vi "P-541 Stage Engine.vi"(0 "Notifier Name":string, 11 "COM Port":string[](array[string])) -> ()   [LabVIEW 2016]
uses:
  Stages Controls/Stage Focus Control.ctl
  Stages Controls/Stage Status.ctl
  Stages Controls/Stage Notifier Element.ctl
  Stages Controls/Stage Actions.ctl
panel:
  out "x-y":dbl[](array[numeric])
  out "On Target?":bool[](array[boolean])
  out "Positions":dbl[](array[numeric])
  in  "Get Position":bool
  in  "ReInitialize":bool
  in  "Error":bool
  out "Status":T1
  in  "Quit":bool
  in  "Focus Control":T2
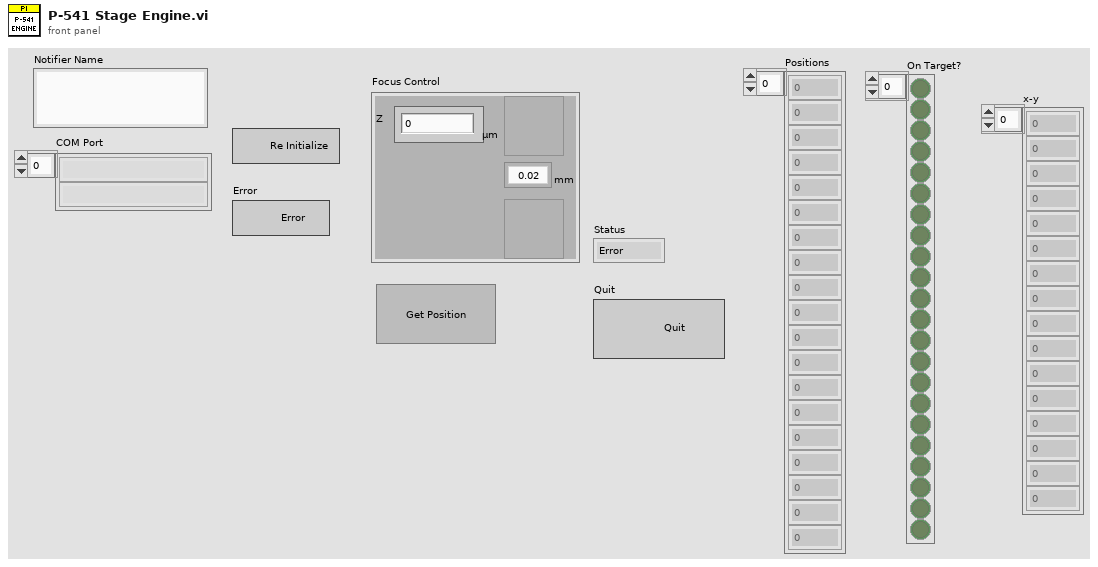
[diagram p1: front panel]
types:
  T1 = typedef "Stage Status.ctl" = enum16{"Error", "Abort", "Busy", "On Target"}
  T2 = typedef "Stage Focus Control.ctl" = cluster{"Focus Step (um)":enum16{"0.02", "0.05", "0.1", "0.5", "1", "2", "5", "10", "20"}, "Focus Up":bool, "Focus Down":bool, "Z ":dbl}
  T3 = typedef "Stage Notifier Element.ctl" = cluster{"Action":T4, "Axis":bool[], "Setpoint":dbl[], "Velocity":dbl, "Cmd Recvd?":bool, "Position":dbl[], "Status":T1, "Misc":variant}
  T4 = typedef "Stage Actions.ctl" = enum16{"Get Position", "MVR", "MOVE", "HALT", "ONTARGET", "ERROR", "REFERENCE", "INIT", "VELOCITY", "STATUS", "EXIT", "HOME", "ZEROPOS", "NANOPOS", "ANALOG", "QUIT"}
  T5 = cluster{"Focus Step (um)":bool, "Focus Up":bool, "Focus Down":bool, "Z ":bool}
  T6 = enum16{"0.02", "0.05", "0.1", "0.5", "1", "2", "5", "10", "20"}
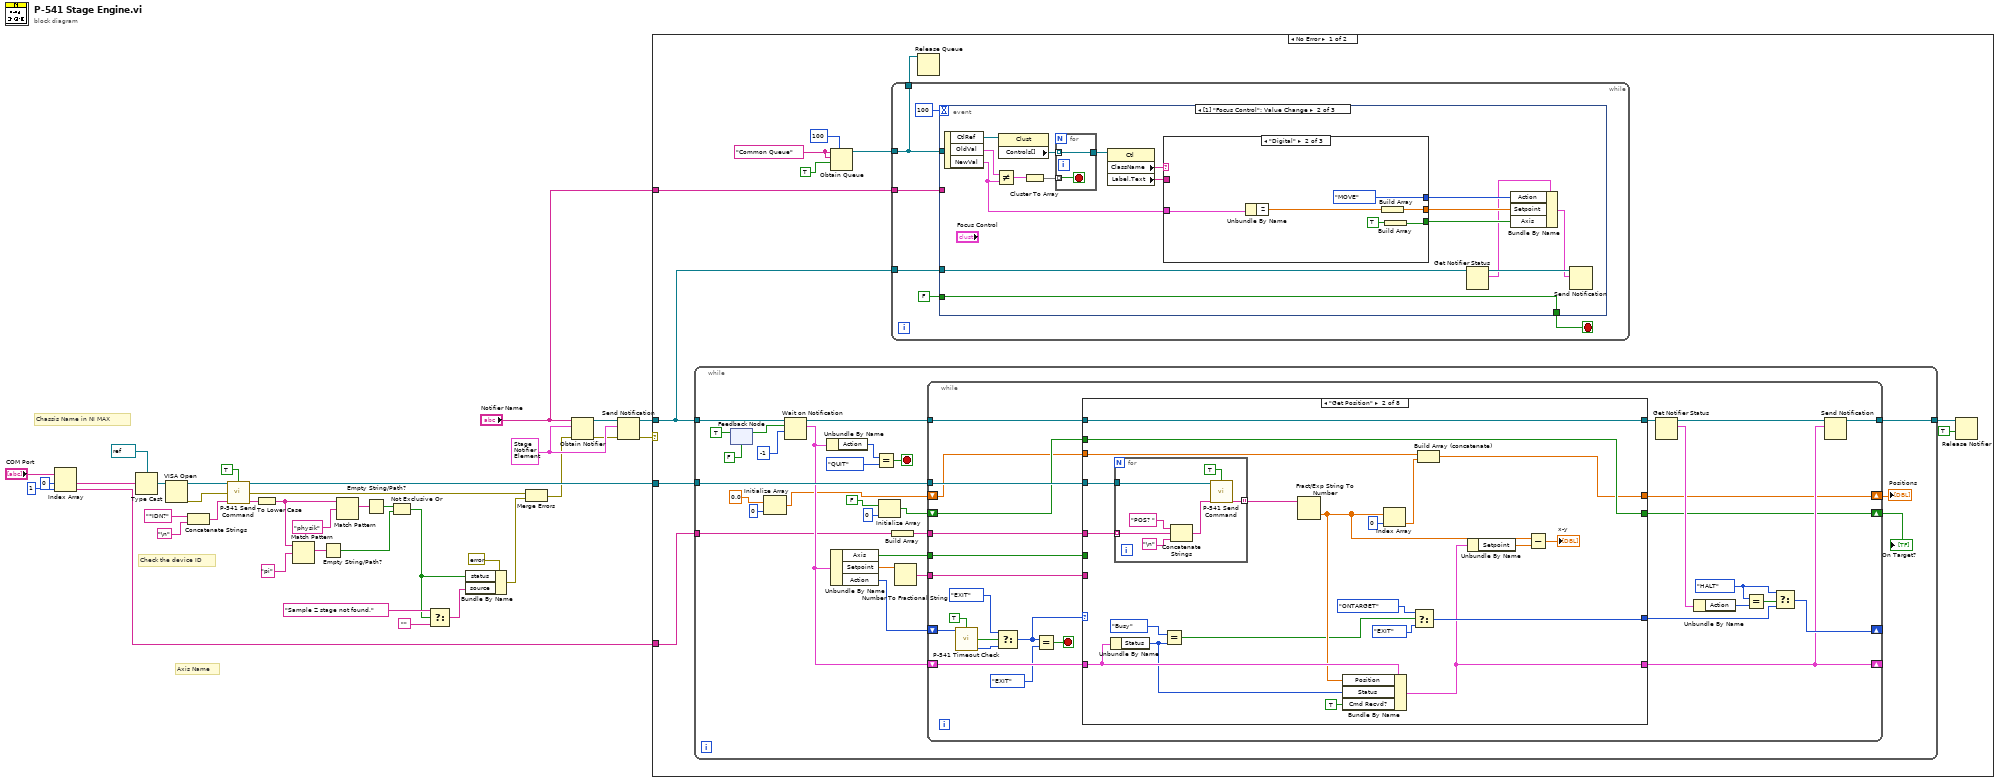
[diagram p0: block diagram]
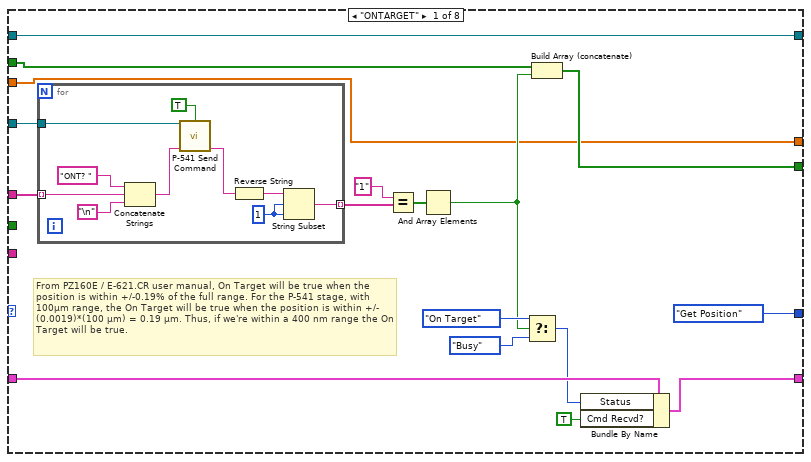
[diagram p2: hidden frame]
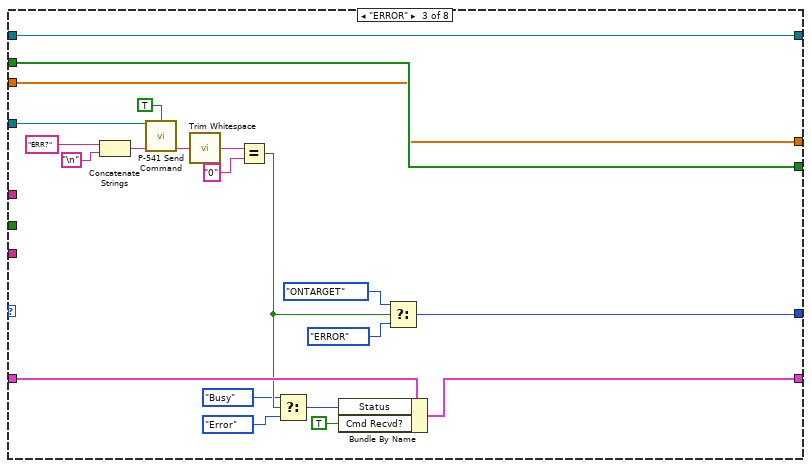
[diagram p3: hidden frame]
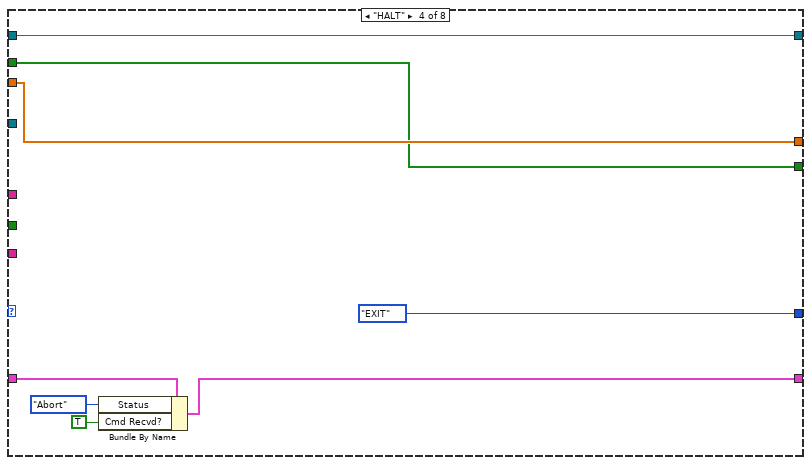
[diagram p4: hidden frame]
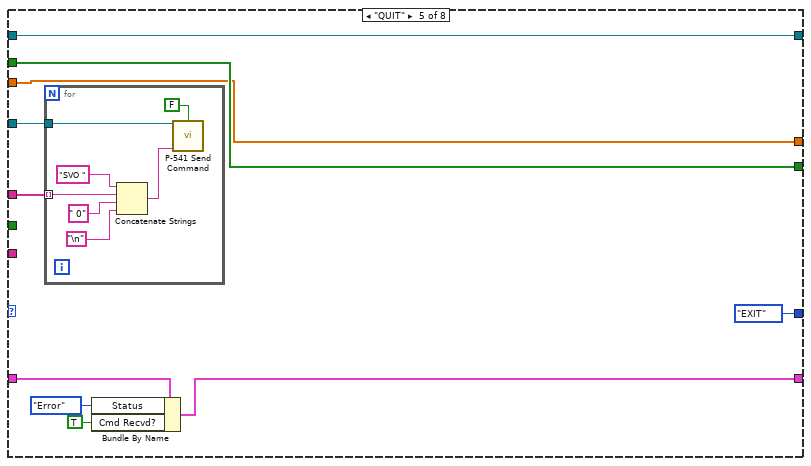
[diagram p5: hidden frame]
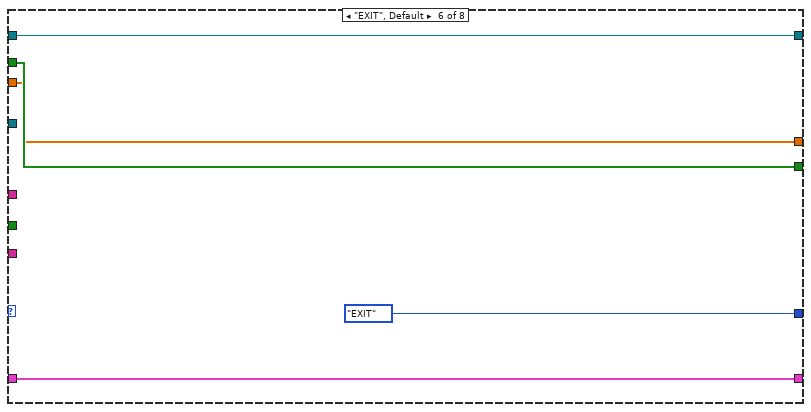
[diagram p6: hidden frame]
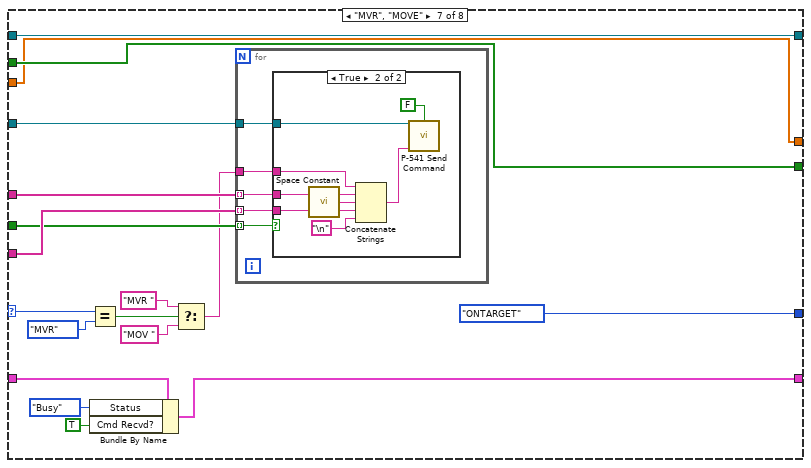
[diagram p7: hidden frame]
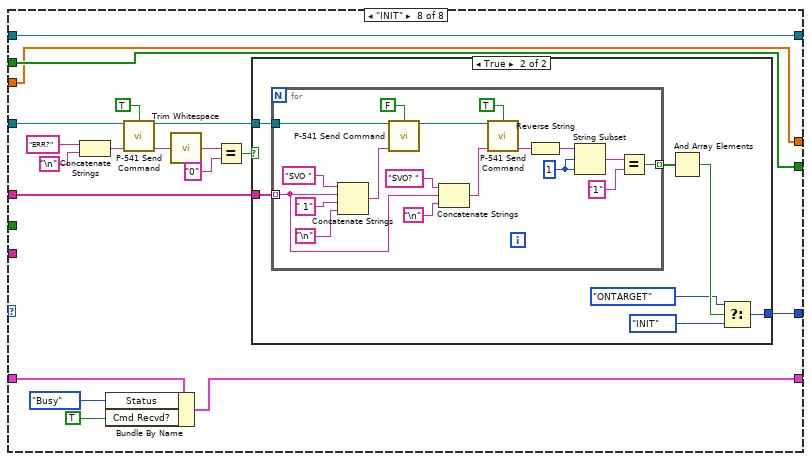
[diagram p9: hidden frame]
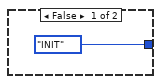
[diagram p10: hidden frame]
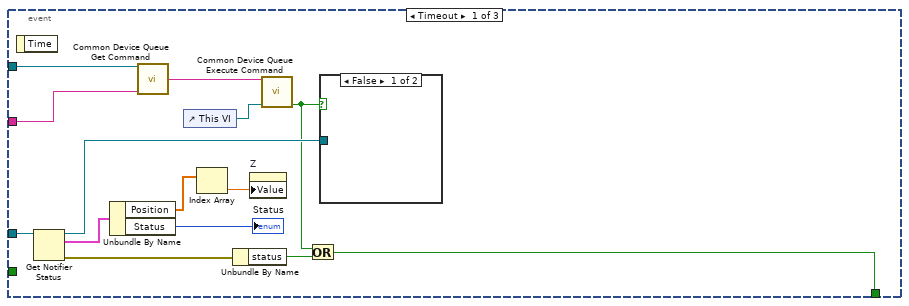
[diagram p11: hidden frame]
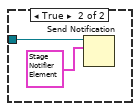
[diagram p12: hidden frame]
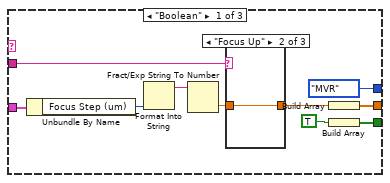
[diagram p13: hidden frame]
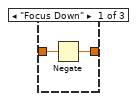
[diagram p14: hidden frame]
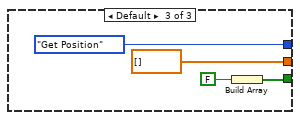
[diagram p16: hidden frame]
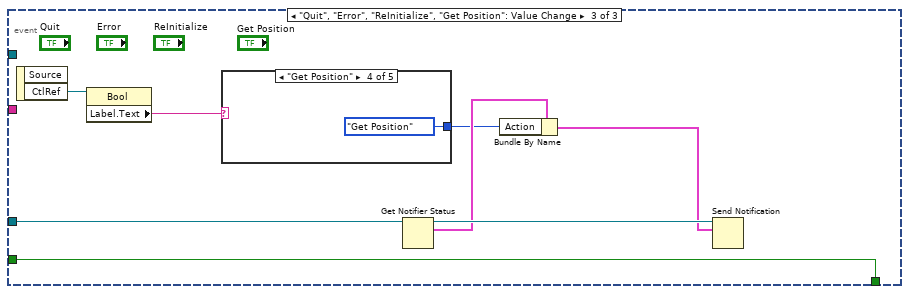
[diagram p17: hidden frame]
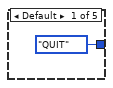
[diagram p18: hidden frame]
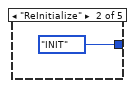
[diagram p19: hidden frame]
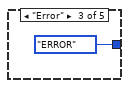
[diagram p20: hidden frame]
diagram:
  w32 = T3 {"Action"=enum."INIT", "Axis"=[], "Setpoint"=[], "Velocity"=0.5, "Cmd Recvd?"=FALSE, "Position"=[], "Status"=enum."Busy", "Misc"=variant} ("Stage Status")
  # "Check the device ID"
  # "Axis Name"
  # "Chassis Name in NI MAX"
  n1 = Index Array(array="COM Port", index #1=0 ("index"), index #2=1 ("index")) -> (element #1=w35:string, element #2=w25:string)
  n2 = Type Cast(type=refnum<visa-resource-name> refnum ("reference out"), x=w35) -> (*(type *) &x=w11:refnum<visa-resource-name>)
  n3 = VISA Open(VISA resource name=w11) -> (VISA resource name=w10:refnum<visa-resource-name>, error out=w7:errorcluster)  [unwired: 4 in]
  n4 = Concatenate Strings("*IDN?" ("string"), "\n") -> (w24:string)
  n5 = call "P-541 Send Command.vi"("VISA Ref"=w10, "Wait for Reply?"=TRUE, "Error In"=w7, "Command"=w24) -> ("VISA Ref Out"=w9:refnum<visa-resource-name>, "Error Out"=w16:errorcluster, "Response"=w18:string)  [unwired: 9 in]
  n6 = To Lower Case(string=w18) -> (all lower case string=w4:string)
  n7 = Match Pattern(string=w4, regular expression="pi" ("string")) -> (match substring=w6:string)  [unwired: 1 in, 3 out]
  n8 = Empty String/Path?(string/path=w6) -> (empty?=w2:bool)
  n9 = Match Pattern(string=w4, regular expression="physik" ("string")) -> (match substring=w20:string)  [unwired: 1 in, 3 out]
  n10 = Empty String/Path?(string/path=w20) -> (empty?=w3:bool)
  n11 = Not Exclusive Or(1:w2, 2:w3) -> (0:w1:bool)
  n12 = Select(t="Sample Z stage not found." ("string"), s=w1, f="") -> (s? t:f=w14:string)
  n13 = Bundle By Name(cluster=errorcluster {"status"=FALSE, "code"=0, "source"=""} ("Error Out"), "status"=w1, "source"=w14) -> (w15:errorcluster)
  n14 = Merge Errors(w16, w15) -> (w8:errorcluster)
  n15 = Obtain Notifier(name (unnamed)="Notifier Name", notification data type=w32, error in (no error)=w8) -> (notifier out=w33:refnum<notifier>, error out=w31:errorcluster)  [unwired: 1 in, 1 out]
  n16 = Send Notification(notification=w32, notifier=w33, error in (no error)=w31) -> (notifier out=w29:refnum<notifier>, error out=w30:errorcluster)
  n17 = case shown="No Error" w30 {
    selector: w30 -> [_ w362]
    tunnel: w29 -> [w41 w364]
    tunnel: w9 -> [w42 w363]
    tunnel: "Notifier Name" -> [w40 _]
    tunnel: w25 -> [w37 _]
    frame No Error {
      w45 = "Common Queue" ("Unique Notifier Name")
      n18 = while {
        tunnel: w41 -> [w72]
        tunnel: w42 -> [w64]
        tunnel: [w57] -> w38
        tunnel: w37 -> [w56]
        stop <- w73 stop-if-true
        n19 = feedback #1(FALSE) -> (w58:bool)
        n20 = feedback-in #1(TRUE) -> ()
        n21 = Initialize Array(0.0, 0 ("dimension size")) -> (w50:dbl[])
        n22 = Wait on Notification(notifier=w72, ignore previous (F)=w58, timeout in ms (-1)=-1) -> (notifier out=w63:refnum<notifier>, notification=w62:T3)  [unwired: 1 in, 2 out]
        n23 = Unbundle By Name(w62) -> ("Action"=w71:T4)
        n24 = Unbundle By Name(w62) -> ("Axis"=w67:bool[], "Setpoint"=w68:dbl[], "Action"=w69:T4)
        n25 = Equal?(x=w71, y=Stage_Actions."QUIT") -> (x = y?=w73:bool)
        n26 = Initialize Array(FALSE, 0 ("dimension size")) -> (w53:bool[])
        n27 = Build Array(w56) -> (w65:string[])
        n28 = Number To Fractional String(number=w68) -> (F-format string=w66:string[])  [unwired: 3 in]
        n29 = while {
          tunnel: w65 -> [w101]
          shift-right: [w82] -> _
          shift-left: w69 -> [w93]
          tunnel: w67 -> [w98]
          tunnel: w66 -> [w99]
          shift-right: [w81] -> _
          shift-left: w62 -> [w97]
          tunnel: w64 -> [w100]
          tunnel: w63 -> [w79]
          tunnel: [w78] -> w57
          shift-right: [w76] -> w48
          shift-left: w53 -> [w77]
          shift-right: [w74] -> w49
          shift-left: w50 -> [w75]
          stop <- w95 stop-if-true
          w84 = Stage_Actions."HALT" ("Action")
          n30 = call "P-541 Timeout Check.vi"("Action"=w93, "User Input?"=TRUE) -> ("Timeout?"=w92:bool, "Action (Dup)"=w91:T4)  [unwired: 12 in]
          n31 = Select(t=Stage_Actions."EXIT" ("y"), s=w92, f=w91) -> (s? t:f=w89:T4)
          n32 = Equal?(x=w89, y=Stage_Actions."EXIT") -> (x = y?=w95:bool)
          n33 = case shown="\"Get Position\"" w89 {
            selector: w89 -> [_ _ _ _ _ _ w216 _]
            tunnel: w101 -> [w118 w149 _ _ w193 _ w225 w257]
            tunnel: w100 -> [w114 w148 w163 _ w194 _ w224 w245]
            tunnel: w99 -> [_ _ _ _ _ _ w223 _]
            tunnel: w98 -> [_ _ _ _ _ _ w222 _]
            tunnel: [Stage_Actions."Get Position" ("y") w146 w172 Stage_Actions."EXIT" ("y") Stage_Actions."EXIT" ("y") Stage_Actions."EXIT" ("y") Stage_Actions."ONTARGET" ("y") w253] -> w83
            tunnel: w97 -> [w111 w144 w167 w181 w191 w207 w219 w254]
            tunnel: [w112 w134 w168 w182 w189 w207 w218 w247] -> w81
            tunnel: [w106 w139 w159 w180 w188 w205 w210 w241] -> w80
            tunnel: w79 -> [w106 w139 w159 w180 w188 w205 w210 w241]
            tunnel: w77 -> [w105 w138 w158 w178 w187 w204 w209 w240]
            tunnel: [w103 w138 w158 w178 w187 w204 w209 w240] -> w76
            tunnel: w75 -> [w102 w136 w157 w179 w186 w203 w208 w239]
            tunnel: [w102 w135 w157 w179 w186 w203 w208 w239] -> w74
            frame "ONTARGET" {
              # "From PZ160E / E-621.CR user manual, On Target will be true when the position is within +/-0.19% of the full range. For the P-541 stage, with 100µm range, the On Target will be true when the position is within +/- (0.0019)*(100 µm) = 0.19 µm. Thus, if we're within a 400 nm range the On Target will be true."
              n34 = for {
                tunnel: w118 -> [w128] mode=indexing
                tunnel: [w127] -> w117 mode=indexing
                tunnel: w114 -> [w121]
                w123 = 1 ("length (rest)")
                n35 = Concatenate Strings("ONT? " ("string"), w128, "\n") -> (w120:string)
                n36 = call "P-541 Send Command.vi"("VISA Ref"=w121, "Wait for Reply?"=TRUE, "Command"=w120) -> ("Response"=w119:string)  [unwired: 10 in, 2 out]
                n37 = Reverse String(1:w119) -> (0:w124:string)
                n38 = String Subset(string=w124, offset (0)=w123, length (rest)=w123) -> (substring=w127:string)
              }
              n39 = Equal?(x="1", y=w117) -> (x = y?=w115:bool[])
              n40 = And Array Elements(Boolean array=w115) -> (logical AND=w104:bool)
              n41 = Select(t=Stage_Status."On Target" ("Status"), s=w104, f=Stage_Status."Busy" ("Status")) -> (s? t:f=w108:T1)
              n42 = Build Array (concatenate)(w105, w104) -> (w103:bool[])
              n43 = Bundle By Name(cluster=w111, "Status"=w108, "Cmd Recvd?"=TRUE) -> (w112:T3)
            }
            frame "Get Position" {
              n44 = Unbundle By Name(w144) -> ("Status"=w142:T1)
              n45 = for {
                tunnel: w149 -> [w156] mode=indexing
                tunnel: w148 -> [w152]
                tunnel: [w150] -> w147 mode=indexing
                n46 = Concatenate Strings("POS? " ("string"), w156, "\n") -> (w151:string)
                n47 = call "P-541 Send Command.vi"("VISA Ref"=w152, "Wait for Reply?"=TRUE, "Command"=w151) -> ("Response"=w150:string)  [unwired: 10 in, 2 out]
              }
              n48 = Equal?(x=Stage_Status."Busy", y=w142) -> (x = y?=w129:bool)
              n49 = Fract/Exp String To Number(string=w147) -> (number=w131:dbl[])  [unwired: 3 in, 1 out]
              n50 = Bundle By Name(cluster=w144, "Position"=w131, "Status"=w142, "Cmd Recvd?"=TRUE) -> (w134:T3)
              n51 = Index Array(array=w131, index=0) -> (element=w133:dbl)
              n52 = Select(t=Stage_Actions."ONTARGET" ("y"), s=w129, f=Stage_Actions."EXIT" ("y")) -> (s? t:f=w146:T4)
              n53 = Build Array (concatenate)(w136, w133) -> (w135:dbl[])
              n54 = Unbundle By Name(w134) -> ("Setpoint"=w132:dbl[])
              n55 = Subtract(x=w131, y=w132) -> (x-y=→"x-y":dbl[])
            }
            frame "ERROR" {
              n56 = Concatenate Strings("ERR?" ("string"), "\n") -> (w162:string)
              n57 = call "P-541 Send Command.vi"("VISA Ref"=w163, "Wait for Reply?"=TRUE, "Command"=w162) -> ("Response"=w161:string)  [unwired: 10 in, 2 out]
              n58 = call <vilib>:"Trim Whitespace.vi"("string"=w161) -> ("trimmed string"=w177:string)  [unwired: 1 in]
              n59 = Equal?(x=w177, y="0") -> (x = y?=w166:bool)
              n60 = Select(t=Stage_Status."Busy" ("Status"), s=w166, f=Stage_Status."Error" ("Status")) -> (s? t:f=w170:T1)
              n61 = Bundle By Name(cluster=w167, "Status"=w170, "Cmd Recvd?"=TRUE) -> (w168:T3)
              n62 = Select(t=Stage_Actions."ONTARGET" ("Action"), s=w166, f=Stage_Actions."ERROR") -> (s? t:f=w172:T4)
            }
            frame "HALT" {
              n63 = Bundle By Name(cluster=w181, "Status"=Stage_Status."Abort", "Cmd Recvd?"=TRUE) -> (w182:T3)
            }
            frame "QUIT" {
              n64 = for {
                tunnel: w193 -> [w199] mode=indexing
                tunnel: w194 -> [w197]
                n65 = Concatenate Strings("SVO " ("write buffer"), w199, " 0" ("string"), "\n") -> (w196:string)
                n66 = call "P-541 Send Command.vi"("VISA Ref"=w197, "Wait for Reply?"=FALSE, "Command"=w196) -> ()  [unwired: 10 in, 3 out]
              }
              n67 = Bundle By Name(cluster=w191, "Status"=Stage_Status."Error", "Cmd Recvd?"=TRUE) -> (w189:T3)
            }
            frame "EXIT", Default {
            }
            frame "MVR", "MOVE" {
              n68 = Equal?(x=w216, y=Stage_Actions."MVR") -> (x = y?=w214:bool)
              n69 = Bundle By Name(cluster=w219, "Status"=Stage_Status."Busy", "Cmd Recvd?"=TRUE) -> (w218:T3)
              n70 = Select(t="MVR ", s=w214, f="MOV ") -> (s? t:f=w211:string)
              n71 = for {
                tunnel: w225 -> [w230] mode=indexing
                tunnel: w223 -> [w229] mode=indexing
                tunnel: w222 -> [w227] mode=indexing
                tunnel: w224 -> [w228]
                tunnel: w211 -> [w226]
                n72 = case shown="True" w227 {
                  tunnel: w230 -> [_ w238]
                  tunnel: w229 -> [_ w235]
                  tunnel: w228 -> [_ w233]
                  tunnel: w226 -> [_ w231]
                  frame False {
                  }
                  frame True {
                    n73 = call <vilib>:"Space Constant.vi"() -> ("String"=w236:string)
                    n74 = Concatenate Strings(w231, w238, w236, w235, "\n") -> (w232:string)
                    n75 = call "P-541 Send Command.vi"("VISA Ref"=w233, "Wait for Reply?"=FALSE, "Command"=w232) -> ()  [unwired: 10 in, 3 out]
                  }
                }
              }
            }
            frame "INIT" {
              n76 = Concatenate Strings("ERR?" ("string"), "\n") -> (w244:string)
              n77 = Bundle By Name(cluster=w254, "Status"=Stage_Status."Busy", "Cmd Recvd?"=TRUE) -> (w247:T3)
              n78 = call "P-541 Send Command.vi"("VISA Ref"=w245, "Wait for Reply?"=TRUE, "Command"=w244) -> ("VISA Ref Out"=w242:refnum<visa-resource-name>, "Response"=w243:string)  [unwired: 10 in, 1 out]
              n79 = call <vilib>:"Trim Whitespace.vi"("string"=w243) -> ("trimmed string"=w250:string)  [unwired: 1 in]
              n80 = Equal?(x=w250, y="0") -> (x = y?=w248:bool)
              n81 = case shown="True" w248 {
                tunnel: w257 -> [_ w265]
                tunnel: [Stage_Actions."INIT" ("y") w261] -> w253
                tunnel: w242 -> [_ w259]
                frame False {
                }
                frame True {
                  n82 = for {
                    tunnel: w265 -> [w276] mode=indexing
                    tunnel: [w274] -> w264 mode=indexing
                    tunnel: w259 -> [w272]
                    w283 = 1 ("length (rest)")
                    n83 = Concatenate Strings("SVO " ("string"), w276, " 1" ("string"), "\n") -> (w271:string)
                    n84 = call "P-541 Send Command.vi"("VISA Ref"=w272, "Wait for Reply?"=FALSE, "Command"=w271) -> ("VISA Ref Out"=w269:refnum<visa-resource-name>)  [unwired: 10 in, 2 out]
                    n85 = Concatenate Strings("SVO? " ("string"), w276, "\n") -> (w268:string)
                    n86 = call "P-541 Send Command.vi"("VISA Ref"=w269, "Wait for Reply?"=TRUE, "Command"=w268) -> ("Response"=w267:string)  [unwired: 10 in, 2 out]
                    n87 = Reverse String(1:w267) -> (0:w282:string)
                    n88 = String Subset(string=w282, offset (0)=w283, length (rest)=w283) -> (substring=w266:string)
                    n89 = Equal?(x=w266, y="1") -> (x = y?=w274:bool)
                  }
                  n90 = And Array Elements(Boolean array=w264) -> (logical AND=w263:bool)
                  n91 = Select(t=Stage_Actions."ONTARGET" ("y"), s=w263, f=Stage_Actions."INIT" ("y")) -> (s? t:f=w261:T4)
                }
              }
            }
          }
          n92 = Get Notifier Status(notifier=w80) -> (notifier out=w88:refnum<notifier>, current notification=w87:T3)  [unwired: 1 in, 3 out]
          n93 = Unbundle By Name(w87) -> ("Action"=w86:T4)
          n94 = Equal?(x=w84, y=w86) -> (x = y?=w85:bool)
          n95 = Select(t=w84, s=w85, f=w83) -> (s? t:f=w82:T4)
          n96 = Send Notification(notification=w81, notifier=w88) -> (notifier out=w78:refnum<notifier>)  [unwired: 1 in, 1 out]
        }
        "Positions" <- w49
        "On Target?" <- w48
      }
      n97 = Obtain Queue(max queue size (-1, unlimited)=100, name (unnamed)=w45, element data type=w45, create if not found? (T)=TRUE) -> (queue out=w44:refnum<queue>)  [unwired: 1 in, 2 out]
      n98 = while {
        tunnel: w41 -> [w287]
        tunnel: w44 -> [w286]
        tunnel: [w286] -> w43
        tunnel: w40 -> [w285]
        stop <- w288 stop-if-true
        n99 = event shown="[1] \"Focus Control\": Value Change" {
          selector: _ -> [_ _ _]
          dyn-events: _ -> [_ _ _]
          timeout: 100 -> [_ _ _]
          tunnel: [w291 w306 w350] -> w288
          tunnel: w287 -> [w302 w311 w356]
          tunnel: w286 -> [w295 _ _]
          tunnel: w285 -> [w290 _ _]
          tunnel: FALSE ("create if not found? (T)") -> [_ w306 w350]
          event Timeout {
            n100 = event-data() -> ()  [unwired: 1 in, 1 out]
            n101 = Get Notifier Status(notifier=w302) -> (notifier out=w294:refnum<notifier>, current notification=w298:T3, error out=w300:errorcluster)  [unwired: 1 in, 2 out]
            n102 = Unbundle By Name(w298) -> ("Position"=w301:dbl[], "Status"=→"Status":T1)
            n103 = call "Common Device Queue Get Command.vi"("Common Queue"=w295, "Notifier Name"=w290) -> ("Command"=w296:string)  [unwired: 12 in, 1 out]
            n104 = control-ref of="This VI"() -> (w297:refnum<vi>)
            n105 = Index Array(array=w301) -> (element=w303:dbl)  [unwired: 1 in]
            n106 = Unbundle By Name(w300) -> ("status"=w293:bool)
            n107 = property on="Z" class="DigNum (strict)"("Value"=w303) -> ()  [unwired: 2 in, 2 out]
            n108 = call "Common Device Queue Execute Command.vi"("Common Command"=w296, "VI Refnum"=w297) -> ("Quit?"=w292:bool)  [unwired: 12 in, 1 out]
            n109 = Or(x=w292, y=w293) -> (x .or. y?=w291:bool)
            n110 = case shown="False" w292 {
              tunnel: w294 -> [_ w305]
              frame False {
              }
              frame True {
                n111 = Send Notification(notification=T3 {"Action"=enum."QUIT", "Axis"=[], "Setpoint"=[], "Velocity"=0.5, "Cmd Recvd?"=FALSE, "Position"=[], "Status"=enum."Error", "Misc"=variant} ("Stage Status"), notifier=w305) -> ()  [unwired: 1 in, 2 out]
              }
            }
          }
          event Value Change {
            n112 = event-data() -> ("CtlRef"=w321:refnum<vi>, "OldVal"=w322:T2, "NewVal"=w315:T2)  [unwired: 1 in]
            n113 = Not Equal?(x=w322, y=w315) -> (x != y?=w320:T5)
            n114 = property class="Clust"(reference=w321) -> ("Controls[]"=w318:refnum<vi>[])  [unwired: 1 in, 2 out]
            n115 = Cluster To Array(cluster=w320) -> (array=w319:bool[])
            n116 = for {
              tunnel: w319 -> [w348] mode=indexing
              tunnel: [w347] -> w317
              tunnel: w318 -> [w347] mode=indexing
              stop <- w348 stop-if-true
            }
            n117 = property class="Ctl"(reference=w317) -> ("ClassName"=w316:string, "Label.Text"=w314:string)  [unwired: 1 in, 2 out]
            n118 = case shown="\"Digital\"" w316 {
              tunnel: w315 -> [w330 w342 _]
              tunnel: w314 -> [w331 _ _]
              tunnel: [w325 w340 dbl[] []] -> w313
              tunnel: [w324 w339 w345] -> w312
              tunnel: [Stage_Actions."MVR" ("Action") Stage_Actions."MOVE" ("Action") Stage_Actions."Get Position" ("Action")] -> w310
              frame "Boolean" {
                n119 = Unbundle By Name(w330) -> ("Focus Step (um)"=w328:T6)
                n120 = Format Into String(w328) -> (resulting string=w329:string)  [unwired: 3 in, 1 out]
                n121 = Fract/Exp String To Number(string=w329) -> (number=w327:dbl)  [unwired: 3 in, 1 out]
                n122 = case shown="\"Focus Up\"" w331 {
                  tunnel: w327 -> [w334 w335 w336]
                  tunnel: [w333 w335 w336] -> w326
                  frame "Focus Down" {
                    n123 = Negate(x=w334) -> (-x=w333:dbl)
                  }
                  frame "Focus Up" {
                  }
                  frame Default {
                  }
                }
                n124 = Build Array(w326) -> (w325:dbl[])
                n125 = Build Array(TRUE) -> (w324:bool[])
              }
              frame "Digital" {
                n126 = Unbundle By Name(w342) -> ("Z"=w341:dbl)
                n127 = Build Array(w341) -> (w340:dbl[])
                n128 = Build Array(TRUE) -> (w339:bool[])
              }
              frame Default {
                n129 = Build Array(FALSE) -> (w345:bool[])
              }
            }
            n130 = Get Notifier Status(notifier=w311) -> (notifier out=w309:refnum<notifier>, current notification=w308:T3)  [unwired: 1 in, 3 out]
            n131 = Bundle By Name(cluster=w308, "Action"=w310, "Setpoint"=w313, "Axis"=w312) -> (w307:T3)
            n132 = Send Notification(notification=w307, notifier=w309) -> ()  [unwired: 1 in, 2 out]
          }
          event "Quit", "Error", "ReInitialize", "Get Position": Value Change {
            n133 = event-data() -> ("CtlRef"=w353:refnum<vi>)  [unwired: 1 in, 1 out]
            n134 = property class="Bool"(reference=w353) -> ("Label.Text"=w352:string)  [unwired: 1 in, 2 out]
            n135 = case shown="\"Get Position\"" w352 {
              tunnel: [Stage_Actions."QUIT" ("Action") Stage_Actions."INIT" ("Action") Stage_Actions."ERROR" ("Action") Stage_Actions."Get Position" ("Action") Stage_Actions."QUIT" ("Action")] -> w351
              frame Default {
              }
              frame "ReInitialize" {
              }
              frame "Error" {
              }
              frame "Get Position" {
              }
              frame "Quit" {
              }
            }
            n136 = Get Notifier Status(notifier=w356) -> (notifier out=w355:refnum<notifier>, current notification=w354:T3)  [unwired: 1 in, 3 out]
            n137 = Bundle By Name(cluster=w354, "Action"=w351) -> (w349:T3)
            n138 = Send Notification(notification=w349, notifier=w355) -> ()  [unwired: 1 in, 2 out]
          }
        }
      }
      n139 = Release Queue(queue=w43) -> ()  [unwired: 2 in, 3 out]
      n140 = Release Notifier(notifier=w38, force destroy? (F)=TRUE) -> ()  [unwired: 1 in, 3 out]
    }
    frame Error {
      n141 = VISA Close(VISA resource name=w363, error in (no error)=w362) -> (error out=w365:errorcluster)
      n142 = Release Notifier(notifier=w364, force destroy? (F)=TRUE, error in (no error)=w365) -> (error out=w370:errorcluster)  [unwired: 2 out]
      n143 = Unbundle By Name(w370) -> ("source"=w367:string)
      n144 = Concatenate Strings("P-541 Stage Error", "\r", w367) -> (w366:string)
      n145 = One Button Dialog(message=w366) -> ()  [unwired: 1 in, 1 out]
    }
  }
